vi "GeoData.vi"() -> ()   [LabVIEW 2017] (continued)
County\tH1\n51467\t19027\tWestside\tIA\tCarroll County\tH1\n51462\t19027\tScranton\tIA\tCarroll County\tH1\n50025\t19027\tAudubon\tIA\tCarroll County\tH1\n51444\t19027\tHalbur\tIA\tCarroll County\tH1\n51451\t19027\tLanesboro\tIA\tCarroll County\tH1\n51436\t19027\tBreda\tIA\tCarroll County\tH1\n51449\t19027\tLake city\tIA\tCarroll County\tH1\n51463\t19027\tTempleton\tIA\tCarroll County\tH1\n50058\t19027\tCoon rapids\tIA\tCarroll County\tH1\n51532\t19029\tElliott\tIA\tCass County\tH1\n50853\t19029\tMassena\tIA\tCass County\tH1\n50843\t19029\tCumberland\tIA\tCass County\tH1\n51552\t19029\tMarne\tIA\tCass County\tH1\n50020\t19029\tAnita\tIA\tCass County\tH1\n50042\t19029\tBrayton\tIA\tCass County\tH1\n50864\t19029\tVillisca\tIA\tCass County\tH1\n51544\t19029\tLewis\tIA\tCass County\tH1\n50022\t19029\tAtlantic\tIA\tCass County\tH1\n51577\t19029\tWalnut\tIA\tCass County\tH1\n51535\t19029\tGriswold\tIA\tCass County\tH1\n50837\t19029\tBridgewater\tIA\tCass County\tH1\n50274\t19029\tWiota\tIA\tCass County\tH1\n52253\t19031\tLisbon\tIA\tCedar County\tH1\n52720\t19031\tAtalissa\tIA\tCedar County\tH1\n52721\t19031\tBennett\tIA\tCedar County\tH1\n52776\t19031\tWest liberty\tIA\tCedar County\tH1\n52323\t19031\tOxford junction\tIA\tCedar County\tH1\n52747\t19031\tDurant\tIA\tCedar County\tH1\n52765\t19031\tNew liberty\tIA\tCedar County\tH1\n52216\t19031\tClarence\tIA\tCedar County\tH1\n52337\t19031\tStanwood\tIA\tCedar County\tH1\n52358\t19031\tWest branch\tIA\tCedar County\tH1\n52255\t19031\tLowden\tIA\tCedar County\tH1\n52333\t19031\tSolon\tIA\tCedar County\tH1\n52772\t19031\tTipton\tIA\tCedar County\tH1\n52778\t19031\tWilton\tIA\tCedar County\tH1\n52320\t19031\tOlin\tIA\tCedar County\tH1\n52760\t19031\tMoscow\tIA\tCedar County\tH1\n52306\t19031\tMechanicsville\tIA\tCedar County\tH1\n52777\t19031\tWheatland\tIA\tCedar County\tH1\n50458\t19033\tNora springs\tIA\tCerro Gordo County\tH1\n50464\t19033\tPlymouth\tIA\tCerro Gordo County\tH1\n50433\t19033\tDougherty\tIA\tCerro Gordo County\tH1\n50467\t19033\tRock falls\tIA\tCerro Gordo County\tH1\n50456\t19033\tManly\tIA\tCerro Gordo County\tH1\n50401\t19033\tMason city\tIA\tCerro Gordo County\tH1\n50469\t19033\tRockwell\tIA\tCerro Gordo County\tH1\n50428\t19033\tClear lake\tIA\tCerro Gordo County\tH1\n50477\t19033\tSwaledale\tIA\tCerro Gordo County\tH1\n50479\t19033\tThornton\tIA\tCerro Gordo County\tH1\n50475\t19033\tSheffield\tIA\tCerro Gordo County\tH1\n50438\t19033\tGarner\tIA\tCerro Gordo County\tH1\n50444\t19033\tHanlontown\tIA\tCerro Gordo County\tH1\n50468\t19033\tRockford\tIA\tCerro Gordo County\tH1\n50482\t19033\tVentura\tIA\tCerro Gordo County\tH1\n50434\t19033\tFertile\tIA\tCerro Gordo County\tH1\n50449\t19033\tKlemme\tIA\tCerro Gordo County\tH1\n50457\t19033\tMeservey\tIA\tCerro Gordo County\tH1\n50402\t19033\tMason city\tIA\tCerro Gordo County\tH1\n51047\t19035\tPeterson\tIA\tCherokee County\tH1\n51046\t19035\tPaullina\tIA\tCherokee County\tH1\n51020\t19035\tGalva\tIA\tCherokee County\tH1\n51048\t19035\tPierson\tIA\tCherokee County\tH1\n51005\t19035\tAurelia\tIA\tCherokee County\tH1\n51002\t19035\tAlta\tIA\tCherokee County\tH1\n51049\t19035\tQuimby\tIA\tCherokee County\tH1\n51037\t19035\tMeriden\tIA\tCherokee County\tH1\n51035\t19035\tMarcus\tIA\tCherokee County\tH1\n51061\t19035\tWashta\tIA\tCherokee County\tH1\n51012\t19035\tCherokee\tIA\tCherokee County\tH1\n51014\t19035\tCleghorn\tIA\tCherokee County\tH1\n51050\t19035\tRemsen\tIA\tCherokee County\tH1\n51025\t19035\tHolstein\tIA\tCherokee County\tH1\n51029\t19035\tLarrabee\tIA\tCherokee County\tH1\n51016\t19035\tCorrectionville\tIA\tCherokee County\tH1\n51022\t19035\tGranville\tIA\tCherokee County\tH1\n51058\t19035\tSutherland\tIA\tCherokee County\tH1\n52132\t19037\tCalmar\tIA\tChickasaw County\tH1\n50645\t19037\tIonia\tIA\tChickasaw County\tH1\n50603\t19037\tAlta vista\tIA\tChickasaw County\tH1\n50659\t19037\tNew hampton\tIA\tChickasaw County\tH1\n50674\t19037\tSumner\tIA\tChickasaw County\tH1\n50630\t19037\tFredericksburg\tIA\tChickasaw County\tH1\n50661\t19037\tNorth washington\tIA\tChickasaw County\tH1\n52144\t19037\tFort atkinson\tIA\tChickasaw County\tH1\n50616\t19037\tCharles city\tIA\tChickasaw County\tH1\n50658\t19037\tNashua\tIA\tChickasaw County\tH1\n52154\t19037\tLawler\tIA\tChickasaw County\tH1\n52171\t19037\tWaucoma\tIA\tChickasaw County\tH1\n50222\t19039\tPeru\tIA\tClarke County\tH1\n50108\t19039\tGrand river\tIA\tClarke County\tH1\n50257\t19039\tTruro\tIA\tClarke County\tH1\n50254\t19039\tThayer\tIA\tClarke County\tH1\n50275\t19039\tWoodburn\tIA\tClarke County\tH1\n50123\t19039\tHumeston\tIA\tClarke County\tH1\n50213\t19039\tOsceola\tIA\tClarke County\tH1\n50264\t19039\tWeldon\tIA\tClarke County\tH1\n50151\t19039\tLucas\tIA\tClarke County\tH1\n50149\t19039\tLorimor\tIA\tClarke County\tH1\n50210\t19039\tNew virginia\tIA\tClarke County\tH1\n50174\t19039\tMurray\tIA\tClarke County\tH1\n51047\t19041\tPeterson\tIA\tClay County\tH1\n51343\t19041\tGreenville\tIA\tClay County\tH1\n50554\t19041\tLaurens\tIA\tClay County\tH1\n51357\t19041\tRoyal\tIA\tClay County\tH1\n51338\t19041\tEverly\tIA\tClay County\tH1\n50565\t19041\tMarathon\tIA\tClay County\tH1\n51346\t19041\tHartley\tIA\tClay County\tH1\n51351\t19041\tMilford\tIA\tClay County\tH1\n51358\t19041\tRuthven\tIA\tClay County\tH1\n51366\t19041\tWebb\tIA\tClay County\tH1\n50515\t19041\tAyrshire\tIA\tClay County\tH1\n51333\t19041\tDickens\tIA\tClay County\tH1\n51341\t19041\tGillett grove\tIA\tClay County\tH1\n51301\t19041\tSpencer\tIA\tClay County\tH1\n51364\t19041\tTerril\tIA\tClay County\tH1\n51340\t19041\tFostoria\tIA\tClay County\tH1\n50585\t19041\tSioux rapids\tIA\tClay County\tH1\n51033\t19041\tLinn grove\tIA\tClay County\tH1\n51058\t19041\tSutherland\tIA\tClay County\tH1\n52035\t19043\tColesburg\tIA\tClayton County\tH1\n52047\t19043\tFarmersburg\tIA\tClayton County\tH1\n52169\t19043\tWadena\tIA\tClayton County\tH1\n52158\t19043\tMarquette\tIA\tClayton County\tH1\n52043\t19043\tElkader\tIA\tClayton County\tH1\n52141\t19043\tElgin\tIA\tClayton County\tH1\n52052\t19043\tGuttenberg\tIA\tClayton County\tH1\n52162\t19043\tPostville\tIA\tClayton County\tH1\n52066\t19043\tNorth buena vista\tIA\tClayton County\tH1\n52076\t19043\tStrawberry point\tIA\tClayton County\tH1\n52048\t19043\tGarber\tIA\tClayton County\tH1\n52053\t19043\tHoly cross\tIA\tClayton County\tH1\n52044\t19043\tElkport\tIA\tClayton County\tH1\n52159\t19043\tMonona\tIA\tClayton County\tH1\n52157\t19043\tMc gregor\tIA\tClayton County\tH1\n50606\t19043\tArlington\tIA\tClayton County\tH1\n52073\t19043\tSherrill\tIA\tClayton County\tH1\n52135\t19043\tClermont\tIA\tClayton County\tH1\n52072\t19043\tSaint olaf\tIA\tClayton County\tH1\n52156\t19043\tLuana\tIA\tClayton County\tH1\n52049\t19043\tGarnavillo\tIA\tClayton County\tH1\n52042\t19043\tEdgewood\tIA\tClayton County\tH1\n52077\t19043\tVolga\tIA\tClayton County\tH1\n52050\t19043\tGreeley\tIA\tClayton County\tH1\n52069\t19045\tPreston\tIA\tClinton County\tH1\n52207\t19045\tBaldwin\tIA\tClinton County\tH1\n52750\t19045\tGoose lake\tIA\tClinton County\tH1\n52730\t19045\tCamanche\tIA\tClinton County\tH1\n52771\t19045\tTeeds grove\tIA\tClinton County\tH1\n52323\t19045\tOxford junction\tIA\tClinton County\tH1\n52742\t19045\tDe witt\tIA\tClinton County\tH1\n52745\t19045\tDixon\tIA\tClinton County\tH1\n52060\t19045\tMaquoketa\tIA\tClinton County\tH1\n52727\t19045\tBryant\tIA\tClinton County\tH1\n52701\t19045\tAndover\tIA\tClinton County\tH1\n52757\t19045\tLow moor\tIA\tClinton County\tH1\n52070\t19045\tSabula\tIA\tClinton County\tH1\n52064\t19045\tMiles\tIA\tClinton County\tH1\n52756\t19045\tLong grove\tIA\tClinton County\tH1\n52309\t19045\tMonmouth\tIA\tClinton County\tH1\n52774\t19045\tWelton\tIA\tClinton County\tH1\n52254\t19045\tLost nation\tIA\tClinton County\tH1\n52732\t19045\tClinton\tIA\tClinton County\tH1\n52731\t19045\tCharlotte\tIA\tClinton County\tH1\n52729\t19045\tCalamus\tIA\tClinton County\tH1\n52037\t19045\tDelmar\tIA\tClinton County\tH1\n52777\t19045\tWheatland\tIA\tClinton County\tH1\n52751\t19045\tGrand mound\tIA\tClinton County\tH1\n51006\t19047\tBattle creek\tIA\tCrawford County\tH1\n51458\t19047\tOdebolt\tIA\tCrawford County\tH1\n51466\t19047\tWall lake\tIA\tCrawford County\tH1\n51465\t19047\tVail\tIA\tCrawford County\tH1\n51441\t19047\tDeloit\tIA\tCrawford County\tH1\n51527\t19047\tDefiance\tIA\tCrawford County\tH1\n51461\t19047\tSchleswig\tIA\tCrawford County\tH1\n51432\t19047\tAspinwall\tIA\tCrawford County\tH1\n51460\t19047\tRicketts\tIA\tCrawford County\tH1\n51455\t19047\tManning\tIA\tCrawford County\tH1\n51034\t19047\tMapleton\tIA\tCrawford County\tH1\n51467\t19047\tWestside\tIA\tCrawford County\tH1\n51529\t19047\tDunlap\tIA\tCrawford County\tH1\n51439\t19047\tCharter oak\tIA\tCrawford County\tH1\n51442\t19047\tDenison\tIA\tCrawford County\tH1\n51454\t19047\tManilla\tIA\tCrawford County\tH1\n51528\t19047\tDow city\tIA\tCrawford County\tH1\n51520\t19047\tArion\tIA\tCrawford County\tH1\n51448\t19047\tKiron\tIA\tCrawford County\tH1\n51444\t19047\tHalbur\tIA\tCrawford County\tH1\n51019\t19047\tDanbury\tIA\tCrawford County\tH1\n51060\t19047\tUte\tIA\tCrawford County\tH1\n51436\t19047\tBreda\tIA\tCrawford County\tH1\n50063\t19049\tDallas center\tIA\tDallas County\tH1\n50220\t19049\tPerry\tIA\tDallas County\tH1\n50109\t19049\tGranger\tIA\tDallas County\tH1\n50233\t19049\tRedfield\tIA\tDallas County\tH1\n50235\t19049\tRippey\tIA\tDallas County\tH1\n50146\t19049\tLinden\tIA\tDallas County\tH1\n50039\t19049\tBouton\tIA\tDallas County\tH1\n50167\t19049\tMinburn\tIA\tDallas County\tH1\n50261\t19049\tVan meter\tIA\tDallas County\tH1\n50263\t19049\tWaukee\tIA\tDallas County\tH1\n50061\t19049\tCumming\tIA\tDallas County\tH1\n50069\t19049\tDe soto\tIA\tDallas County\tH1\n50070\t19049\tDexter\tIA\tDallas County\tH1\n50325\t19049\tClive\tIA\tDallas County\tH1\n50128\t19049\tJamaica\tIA\tDallas County\tH1\n50003\t19049\tAdel\tIA\tDallas County\tH1\n50156\t19049\tMadrid\tIA\tDallas County\tH1\n50066\t19049\tDawson\tIA\tDallas County\tH1\n50216\t19049\tPanora\tIA\tDallas County\tH1\n50276\t19049\tWoodward\tIA\tDallas County\tH1\n50111\t19049\tGrimes\tIA\tDallas County\tH1\n50323\t19049\tUrbandale\tIA\tDallas County\tH1\n50277\t19049\tYale\tIA\tDallas County\tH1\n50072\t19049\tEarlham\tIA\tDallas County\tH1\n50038\t19049\tBooneville\tIA\tDallas County\tH1\n50266\t19049\tWest des moines\tIA\tDallas County\tH1\n52560\t19051\tFloris\tIA\tDavis County\tH1\n52570\t19051\tMilton\tIA\tDavis County\tH1\n52584\t19051\tPulaski\tIA\tDavis County\tH1\n52551\t19051\tDouds\tIA\tDavis County\tH1\n52552\t19051\tDrakesville\tIA\tDavis County\tH1\n52536\t19051\tBlakesburg\tIA\tDavis County\tH1\n52588\t19051\tSelma\tIA\tDavis County\tH1\n52554\t19051\tEldon\tIA\tDavis County\tH1\n52572\t19051\tMoulton\tIA\tDavis County\tH1\n52537\t19051\tBloomfield\tIA\tDavis County\tH1\n52594\t19051\tUnionville\tIA\tDavis County\tH1\n50108\t19053\tGrand river\tIA\tDecatur County\tH1\n50147\t19053\tLineville\tIA\tDecatur County\tH1\n50067\t19053\tDecatur\tIA\tDecatur County\tH1\n50140\t19053\tLamoni\tIA\tDecatur County\tH1\n50065\t19053\tDavis city\tIA\tDecatur County\tH1\n50123\t19053\tHumeston\tIA\tDecatur County\tH1\n50264\t19053\tWeldon\tIA\tDecatur County\tH1\n50262\t19053\tVan wert\tIA\tDecatur County\tH1\n50133\t19053\tKellerton\tIA\tDecatur County\tH1\n50103\t19053\tGarden grove\tIA\tDecatur County\tH1\n50144\t19053\tLeon\tIA\tDecatur County\tH1\n52065\t19055\tNew vienna\tIA\tDelaware County\tH1\n52035\t19055\tColesburg\tIA\tDelaware County\tH1\n52237\t19055\tHopkinton\tIA\tDelaware County\tH1\n52057\t19055\tManchester\tIA\tDelaware County\tH1\n52223\t19055\tDelhi\tIA\tDelaware County\tH1\n52330\t19055\tRyan\tIA\tDelaware County\tH1\n50650\t19055\tLamont\tIA\tDelaware County\tH1\n52036\t19055\tDelaware\tIA\tDelaware County\tH1\n52041\t19055\tEarlville\tIA\tDelaware County\tH1\n52076\t19055\tStrawberry point\tIA\tDelaware County\tH1\n52310\t19055\tMonticello\tIA\tDelaware County\tH1\n52038\t19055\tDundee\tIA\tDelaware County\tH1\n52078\t19055\tWorthington\tIA\tDelaware County\tH1\n50654\t19055\tMasonville\tIA\tDelaware County\tH1\n52040\t19055\tDyersville\tIA\tDelaware County\tH1\n52042\t19055\tEdgewood\tIA\tDelaware County\tH1\n52218\t19055\tCoggon\tIA\tDelaware County\tH1\n52050\t19055\tGreeley\tIA\tDelaware County\tH1\n52640\t19057\tMorning sun\tIA\tDes Moines County\tH1\n52646\t19057\tOakville\tIA\tDes Moines County\tH1\n52623\t19057\tDanville\tIA\tDes Moines County\tH1\n52638\t19057\tMiddletown\tIA\tDes Moines County\tH1\n52601\t19057\tBurlington\tIA\tDes Moines County\tH1\n52650\t19057\tSperry\tIA\tDes Moines County\tH1\n52655\t19057\tWest burlington\tIA\tDes Moines County\tH1\n52637\t19057\tMediapolis\tIA\tDes Moines County\tH1\n52645\t19057\tNew london\tIA\tDes Moines County\tH1\n52644\t19057\tMount union\tIA\tDes Moines County\tH1\n52658\t19057\tWever\tIA\tDes Moines County\tH1\n52660\t19057\tYarmouth\tIA\tDes Moines County\tH1\n51347\t19059\tLake park\tIA\tDickinson County\tH1\n51355\t19059\tOkoboji\tIA\tDickinson County\tH1\n51338\t19059\tEverly\tIA\tDickinson County\tH1\n51351\t19059\tMilford\tIA\tDickinson County\tH1\n51331\t19059\tArnolds park\tIA\tDickinson County\tH1\n51333\t19059\tDickens\tIA\tDickinson County\tH1\n51301\t19059\tSpencer\tIA\tDickinson County\tH1\n51345\t19059\tHarris\tIA\tDickinson County\tH1\n51364\t19059\tTerril\tIA\tDickinson County\tH1\n51360\t19059\tSpirit lake\tIA\tDickinson County\tH1\n51334\t19059\tEstherville\tIA\tDickinson County\tH1\n51363\t19059\tSuperior\tIA\tDickinson County\tH1\n52033\t19061\tCascade\tIA\tDubuque County\tH1\n52065\t19061\tNew vienna\tIA\tDubuque County\tH1\n52054\t19061\tLa motte\tIA\tDubuque County\tH1\n52002\t19061\tDubuque\tIA\tDubuque County\tH1\n52003\t19061\tDubuque\tIA\tDubuque County\tH1\n52039\t19061\tDurango\tIA\tDubuque County\tH1\n52045\t19061\tEpworth\tIA\tDubuque County\tH1\n52237\t19061\tHopkinton\tIA\tDubuque County\tH1\n52079\t19061\tZwingle\tIA\tDubuque County\tH1\n52056\t19061\tLuxemburg\tIA\tDubuque County\tH1\n52046\t19061\tFarley\tIA\tDubuque County\tH1\n52052\t19061\tGuttenberg\tIA\tDubuque County\tH1\n52066\t19061\tNorth buena vista\tIA\tDubuque County\tH1\n52053\t19061\tHoly cross\tIA\tDubuque County\tH1\n52099\t19061\tDubuque\tIA\tDubuque County\tH1\n52032\t19061\tBernard\tIA\tDubuque County\tH1\n52073\t19061\tSherrill\tIA\tDubuque County\tH1\n52078\t19061\tWorthington\tIA\tDubuque County\tH1\n52001\t19061\tDubuque\tIA\tDubuque County\tH1\n52068\t19061\tPeosta\tIA\tDubuque County\tH1\n52031\t19061\tBellevue\tIA\tDubuque County\tH1\n52040\t19061\tDyersville\tIA\tDubuque County\tH1\n52004\t19061\tDubuque\tIA\tDubuque County\tH1\n51365\t19063\tWallingford\tIA\tEmmet County\tH1\n50514\t19063\tArmstrong\tIA\tEmmet County\tH1\n50578\t19063\tRingsted\tIA\tEmmet County\tH1\n51342\t19063\tGraettinger\tIA\tEmmet County\tH1\n50539\t19063\tFenton\tIA\tEmmet County\tH1\n51364\t19063\tTerril\tIA\tEmmet County\tH1\n51334\t19063\tEstherville\tIA\tEmmet County\tH1\n50531\t19063\tDolliver\tIA\tEmmet County\tH1\n50655\t19065\tMaynard\tIA\tFayette County\tH1\n50662\t19065\tOelwein\tIA\tFayette County\tH1\n50681\t19065\tWestgate\tIA\tFayette County\tH1\n52147\t19065\tHawkeye\tIA\tFayette County\tH1\n52169\t19065\tWadena\tIA\tFayette County\tH1\n52141\t19065\tElgin\tIA\tFayette County\tH1\n52164\t19065\tRandalia\tIA\tFayette County\tH1\n50650\t19065\tLamont\tIA\tFayette County\tH1\n52161\t19065\tOssian\tIA\tFayette County\tH1\n52175\t19065\tWest union\tIA\tFayette County\tH1\n52162\t19065\tPostville\tIA\tFayette County\tH1\n50674\t19065\tSumner\tIA\tFayette County\tH1\n52076\t19065\tStrawberry point\tIA\tFayette County\tH1\n50664\t19065\tOran\tIA\tFayette County\tH1\n50629\t19065\tFairbank\tIA\tFayette County\tH1\n52142\t19065\tFayette\tIA\tFayette County\tH1\n50606\t19065\tArlington\tIA\tFayette County\tH1\n52133\t19065\tCastalia\tIA\tFayette County\tH1\n52135\t19065\tClermont\tIA\tFayette County\tH1\n52144\t19065\tFort atkinson\tIA\tFayette County\tH1\n50607\t19065\tAurora\tIA\tFayette County\tH1\n50671\t19065\tStanley\tIA\tFayette County\tH1\n52171\t19065\tWaucoma\tIA\tFayette County\tH1\n52166\t19065\tSaint lucas\tIA\tFayette County\tH1\n50458\t19067\tNora springs\tIA\tFloyd County\tH1\n50433\t19067\tDougherty\tIA\tFloyd County\tH1\n50461\t19067\tOsage\tIA\tFloyd County\tH1\n50636\t19067\tGreene\tIA\tFloyd County\tH1\n50653\t19067\tMarble rock\tIA\tFloyd County\tH1\n50620\t19067\tColwell\tIA\tFloyd County\tH1\n50645\t19067\tIonia\tIA\tFloyd County\tH1\n50471\t19067\tRudd\tIA\tFloyd County\tH1\n50619\t19067\tClarksville\tIA\tFloyd County\tH1\n50468\t19067\tRockford\tIA\tFloyd County\tH1\n50435\t19067\tFloyd\tIA\tFloyd County\tH1\n50460\t19067\tOrchard\tIA\tFloyd County\tH1\n50616\t19067\tCharles city\tIA\tFloyd County\tH1\n50658\t19067\tNashua\tIA\tFloyd County\tH1\n50071\t19069\tDows\tIA\tFranklin County\tH1\n50433\t19069\tDougherty\tIA\tFranklin County\tH1\n50625\t19069\tDumont\tIA\tFranklin County\tH1\n50633\t19069\tGeneva\tIA\tFranklin County\tH1\n50126\t19069\tIowa falls\tIA\tFranklin County\tH1\n50479\t19069\tThornton\tIA\tFranklin County\tH1\n50605\t19069\tAredale\tIA\tFranklin County\tH1\n50475\t19069\tSheffield\tIA\tFranklin County\tH1\n50470\t19069\tRowan\tIA\tFranklin County\tH1\n50452\t19069\tLatimer\tIA\tFranklin County\tH1\n50601\t19069\tAckley\tIA\tFranklin County\tH1\n50006\t19069\tAlden\tIA\tFranklin County\tH1\n50420\t19069\tAlexander\tIA\tFranklin County\tH1\n50427\t19069\tChapin\tIA\tFranklin County\tH1\n50441\t19069\tHampton\tIA\tFranklin County\tH1\n50457\t19069\tMeservey\tIA\tFranklin County\tH1\n50041\t19069\tBradford\tIA\tFranklin County\tH1\n50227\t19069\tPopejoy\tIA\tFranklin County\tH1\n50431\t19069\tCoulter\tIA\tFranklin County\tH1\n51647\t19071\tNorthboro\tIA\tFremont County\tH1\n51551\t19071\tMalvern\tIA\tFremont County\tH1\n51640\t19071\tHamburg\tIA\tFremont County\tH1\n51648\t19071\tPercival\tIA\tFremont County\tH1\n51650\t19071\tRiverton\tIA\tFremont County\tH1\n51603\t19071\tShenandoah\tIA\tFremont County\tH1\n51601\t19071\tShenandoah\tIA\tFremont County\tH1\n51654\t19071\tThurman\tIA\tFremont County\tH1\n51649\t19071\tRandolph\tIA\tFremont County\tH1\n51653\t19071\tTabor\tIA\tFremont County\tH1\n51639\t19071\tFarragut\tIA\tFremont County\tH1\n51652\t19071\tSidney\tIA\tFremont County\tH1\n51645\t19071\tImogene\tIA\tFremont County\tH1\n50220\t19073\tPerry\tIA\tGreene County\tH1\n50543\t19073\tGowrie\tIA\tGreene County\tH1\n50064\t19073\tDana\tIA\tGreene County\tH1\n50235\t19073\tRippey\tIA\tGreene County\tH1\n50026\t19073\tBagley\tIA\tGreene County\tH1\n51453\t19073\tLohrville\tIA\tGreene County\tH1\n50050\t19073\tChurdan\tIA\tGreene County\tH1\n51443\t19073\tGlidden\tIA\tGreene County\tH1\n50029\t19073\tBayard\tIA\tGreene County\tH1\n50128\t19073\tJamaica\tIA\tGreene County\tH1\n51462\t19073\tScranton\tIA\tGreene County\tH1\n50544\t19073\tHarcourt\tIA\tGreene County\tH1\n50217\t19073\tPaton\tIA\tGreene County\tH1\n50107\t19073\tGrand junction\tIA\tGreene County\tH1\n51449\t19073\tLake city\tIA\tGreene County\tH1\n50129\t19073\tJefferson\tIA\tGreene County\tH1\n50058\t19073\tCoon rapids\tIA\tGreene County\tH1\n50059\t19073\tCooper\tIA\tGreene County\tH1\n50638\t19075\tGrundy center\tIA\tGrundy County\tH1\n50148\t19075\tLiscomb\tIA\tGrundy County\tH1\n50621\t19075\tConrad\tIA\tGrundy County\tH1\n50613\t19075\tCedar falls\tIA\tGrundy County\tH1\n50657\t19075\tMorrison\tIA\tGrundy County\tH1\n50672\t19075\tSteamboat rock\tIA\tGrundy County\tH1\n50669\t19075\tReinbeck\tIA\tGrundy County\tH1\n50609\t19075\tBeaman\tIA\tGrundy County\tH1\n50269\t19075\tWhitten\tIA\tGrundy County\tH1\n50673\t19075\tStout\tIA\tGrundy County\tH1\n50601\t19075\tAckley\tIA\tGrundy County\tH1\n50680\t19075\tWellsburg\tIA\tGrundy County\tH1\n50665\t19075\tParkersburg\tIA\tGrundy County\tH1\n50624\t19075\tDike\tIA\tGrundy County\tH1\n50642\t19075\tHolland\tIA\tGrundy County\tH1\n50258\t19075\tUnion\tIA\tGrundy County\tH1\n50627\t19075\tEldora\tIA\tGrundy County\tH1\n50604\t19075\tAplington\tIA\tGrundy County\tH1\n50660\t19075\tNew hartford\tIA\tGrundy County\tH1\n50643\t19075\tHudson\tIA\tGrundy County\tH1\n50002\t19077\tAdair\tIA\tGuthrie County\tH1\n50076\t19077\tExira\tIA\tGuthrie County\tH1\n50233\t19077\tRedfield\tIA\tGuthrie County\tH1\n50115\t19077\tGuthrie center\tIA\tGuthrie County\tH1\n50146\t19077\tLinden\tIA\tGuthrie County\tH1\n50048\t19077\tCasey\tIA\tGuthrie County\tH1\n50026\t19077\tBagley\tIA\tGuthrie County\tH1\n50250\t19077\tStuart\tIA\tGuthrie County\tH1\n50070\t19077\tDexter\tIA\tGuthrie County\tH1\n50020\t19077\tAnita\tIA\tGuthrie County\tH1\n50029\t19077\tBayard\tIA\tGuthrie County\tH1\n50128\t19077\tJamaica\tIA\tGuthrie County\tH1\n50216\t19077\tPanora\tIA\tGuthrie County\tH1\n50164\t19077\tMenlo\tIA\tGuthrie County\tH1\n50277\t19077\tYale\tIA\tGuthrie County\tH1\n50129\t19077\tJefferson\tIA\tGuthrie County\tH1\n50058\t19077\tCoon rapids\tIA\tGuthrie County\tH1\n50236\t19079\tRoland\tIA\tHamilton County\tH1\n50230\t19079\tRadcliffe\tIA\tHamilton County\tH1\n50246\t19079\tStanhope\tIA\tHamilton County\tH1\n50231\t19079\tRandall\tIA\tHamilton County\tH1\n50034\t19079\tBlairsburg\tIA\tHamilton County\tH1\n50132\t19079\tKamrar\tIA\tHamilton County\tH1\n50595\t19079\tWebster city\tIA\tHamilton County\tH1\n50599\t19079\tWoolstock\tIA\tHamilton County\tH1\n50036\t19079\tBoone\tIA\tHamilton County\tH1\n50249\t19079\tStratford\tIA\tHamilton County\tH1\n50271\t19079\tWilliams\tIA\tHamilton County\tH1\n50006\t19079\tAlden\tIA\tHamilton County\tH1\n50075\t19079\tEllsworth\tIA\tHamilton County\tH1\n50248\t19079\tStory city\tIA\tHamilton County\tH1\n50532\t19079\tDuncombe\tIA\tHamilton County\tH1\n50130\t19079\tJewell\tIA\tHamilton County\tH1\n50447\t19081\tKanawha\tIA\tHancock County\tH1\n50483\t19081\tWesley\tIA\tHancock County\tH1\n50438\t19081\tGarner\tIA\tHancock County\tH1\n50423\t19081\tBritt\tIA\tHancock County\tH1\n50482\t19081\tVentura\tIA\tHancock County\tH1\n50439\t19081\tGoodell\tIA\tHancock County\tH1\n50484\t19081\tWoden\tIA\tHancock County\tH1\n50421\t19081\tBelmond\tIA\tHancock County\tH1\n50432\t19081\tCrystal lake\tIA\tHancock County\tH1\n50436\t19081\tForest city\tIA\tHancock County\tH1\n50449\t19081\tKlemme\tIA\tHancock County\tH1\n50457\t19081\tMeservey\tIA\tHancock County\tH1\n50430\t19081\tCorwith\tIA\tHancock County\tH1\n50206\t19083\tNew providence\tIA\tHardin County\tH1\n50259\t19083\tGifford\tIA\tHardin County\tH1\n50230\t19083\tRadcliffe\tIA\tHardin County\tH1\n50126\t19083\tIowa falls\tIA\tHardin County\tH1\n50122\t19083\tHubbard\tIA\tHardin County\tH1\n50672\t19083\tSteamboat rock\tIA\tHardin County\tH1\n50271\t19083\tWilliams\tIA\tHardin County\tH1\n50269\t19083\tWhitten\tIA\tHardin County\tH1\n50601\t19083\tAckley\tIA\tHardin County\tH1\n50006\t19083\tAlden\tIA\tHardin County\tH1\n50102\t19083\tGarden city\tIA\tHardin County\tH1\n50258\t19083\tUnion\tIA\tHardin County\tH1\n50154\t19083\tMc callsburg\tIA\tHardin County\tH1\n50627\t19083\tEldora\tIA\tHardin County\tH1\n50227\t19083\tPopejoy\tIA\tHardin County\tH1\n51550\t19085\tMagnolia\tIA\tHarrison County\tH1\n51557\t19085\tMondamin\tIA\tHarrison County\tH1\n51564\t19085\tPisgah\tIA\tHarrison County\tH1\n51563\t19085\tPersia\tIA\tHarrison County\tH1\n51579\t19085\tWoodbine\tIA\tHarrison County\tH1\n51545\t19085\tLittle sioux\tIA\tHarrison County\tH1\n51555\t19085\tMissouri valley\tIA\tHarrison County\tH1\n51562\t19085\tPanama\tIA\tHarrison County\tH1\n51523\t19085\tBlencoe\tIA\tHarrison County\tH1\n51529\t19085\tDunlap\tIA\tHarrison County\tH1\n51565\t19085\tPortsmouth\tIA\tHarrison County\tH1\n51530\t19085\tEarling\tIA\tHarrison County\tH1\n51559\t19085\tNeola\tIA\tHarrison County\tH1\n51556\t19085\tModale\tIA\tHarrison County\tH1\n51546\t19085\tLogan\tIA\tHarrison County\tH1\n51570\t19085\tShelby\tIA\tHarrison County\tH1\n51558\t19085\tMoorhead\tIA\tHarrison County\tH1\n52656\t19087\tWest point\tIA\tHenry County\tH1\n52641\t19087\tMount pleasant\tIA\tHenry County\tH1\n52659\t19087\tWinfield\tIA\tHenry County\tH1\n52621\t19087\tCrawfordsville\tIA\tHenry County\tH1\n52647\t19087\tOlds\tIA\tHenry County\tH1\n52620\t19087\tBonaparte\tIA\tHenry County\tH1\n52652\t19087\tSwedesburg\tIA\tHenry County\tH1\n52630\t19087\tHillsboro\tIA\tHenry County\tH1\n52623\t19087\tDanville\tIA\tHenry County\tH1\n52635\t19087\tLockridge\tIA\tHenry County\tH1\n52637\t19087\tMediapolis\tIA\tHenry County\tH1\n52645\t19087\tNew london\tIA\tHenry County\tH1\n52644\t19087\tMount union\tIA\tHenry County\tH1\n52649\t19087\tSalem\tIA\tHenry County\tH1\n52654\t19087\tWayland\tIA\tHenry County\tH1\n50628\t19089\tElma\tIA\tHoward County\tH1\n52132\t19089\tCalmar\tIA\tHoward County\tH1\n52163\t19089\tProtivin\tIA\tHoward County\tH1\n50603\t19089\tAlta vista\tIA\tHoward County\tH1\n50466\t19089\tRiceville\tIA\tHoward County\tH1\n50659\t19089\tNew hampton\tIA\tHoward County\tH1\n52136\t19089\tCresco\tIA\tHoward County\tH1\n52134\t19089\tChester\tIA\tHoward County\tH1\n52155\t19089\tLime springs\tIA\tHoward County\tH1\n52154\t19089\tLawler\tIA\tHoward County\tH1\n52171\t19089\tWaucoma\tIA\tHoward County\tH1\n50519\t19091\tBode\tIA\tHumboldt County\tH1\n50548\t19091\tHumboldt\tIA\tHumboldt County\tH1\n50570\t19091\tOttosen\tIA\tHumboldt County\tH1\n50516\t19091\tBadger\tIA\tHumboldt County\tH1\n50558\t19091\tLivermore\tIA\tHumboldt County\tH1\n50560\t19091\tLu verne\tIA\tHumboldt County\tH1\n50520\t19091\tBradgate\tIA\tHumboldt County\tH1\n50541\t19091\tGilmore city\tIA\tHumboldt County\tH1\n50542\t19091\tGoldfield\tIA\tHumboldt County\tH1\n50577\t19091\tRenwick\tIA\tHumboldt County\tH1\n50524\t19091\tClare\tIA\tHumboldt County\tH1\n50529\t19091\tDakota city\tIA\tHumboldt County\tH1\n50591\t19091\tThor\tIA\tHumboldt County\tH1\n50582\t19091\tRutland\tIA\tHumboldt County\tH1\n50533\t19091\tEagle grove\tIA\tHumboldt County\tH1\n50545\t19091\tHardy\tIA\tHumboldt County\tH1\n50597\t19091\tWest bend\tIA\tHumboldt County\tH1\n50430\t19091\tCorwith\tIA\tHumboldt County\tH1\n51006\t19093\tBattle creek\tIA\tIda County\tH1\n51020\t19093\tGalva\tIA\tIda County\tH1\n51445\t19093\tIda grove\tIA\tIda County\tH1\n51461\t19093\tSchleswig\tIA\tIda County\tH1\n51431\t19093\tArthur\tIA\tIda County\tH1\n51053\t19093\tSchaller\tIA\tIda County\tH1\n51061\t19093\tWashta\tIA\tIda County\tH1\n51448\t19093\tKiron\tIA\tIda County\tH1\n51019\t19093\tDanbury\tIA\tIda County\tH1\n51025\t19093\tHolstein\tIA\tIda County\tH1\n51016\t19093\tCorrectionville\tIA\tIda County\tH1\n51018\t19093\tCushing\tIA\tIda County\tH1\n52361\t19095\tWilliamsburg\tIA\tIowa County\tH1\n50136\t19095\tKeswick\tIA\tIowa County\tH1\n52232\t19095\tHartwick\tIA\tIowa County\tH1\n52236\t19095\tHomestead\tIA\tIowa County\tH1\n52204\t19095\tAmana\tIA\tIowa County\tH1\n52222\t19095\tDeep river\tIA\tIowa County\tH1\n52355\t19095\tWebster\tIA\tIowa County\tH1\n52301\t19095\tMarengo\tIA\tIowa County\tH1\n52347\t19095\tVictor\tIA\tIowa County\tH1\n52322\t19095\tOxford\tIA\tIowa County\tH1\n52209\t19095\tBlairstown\tIA\tIowa County\tH1\n52203\t19095\tAmana\tIA\tIowa County\tH1\n52318\t19095\tNorway\tIA\tIowa County\tH1\n52221\t19095\tGuernsey\tIA\tIowa County\tH1\n52316\t19095\tNorth english\tIA\tIowa County\tH1\n52307\t19095\tMiddle amana\tIA\tIowa County\tH1\n52208\t19095\tBelle plaine\tIA\tIowa County\tH1\n52356\t19095\tWellman\tIA\tIowa County\tH1\n52334\t19095\tSouth amana\tIA\tIowa County\tH1\n52308\t19095\tMillersburg\tIA\tIowa County\tH1\n52220\t19095\tConroy\tIA\tIowa County\tH1\n52325\t19095\tParnell\tIA\tIowa County\tH1\n52251\t19095\tLadora\tIA\tIowa County\tH1\n52069\t19097\tPreston\tIA\tJackson County\tH1\n52207\t19097\tBaldwin\tIA\tJackson County\tH1\n52054\t19097\tLa motte\tIA\tJackson County\tH1\n52030\t19097\tAndrew\tIA\tJackson County\tH1\n52079\t19097\tZwingle\tIA\tJackson County\tH1\n52060\t19097\tMaquoketa\tIA\tJackson County\tH1\n52071\t19097\tSaint donatus\tIA\tJackson County\tH1\n52070\t19097\tSabula\tIA\tJackson County\tH1\n52064\t19097\tMiles\tIA\tJackson County\tH1\n52074\t19097\tSpragueville\tIA\tJackson County\tH1\n52309\t19097\tMonmouth\tIA\tJackson County\tH1\n52032\t19097\tBernard\tIA\tJackson County\tH1\n52731\t19097\tCharlotte\tIA\tJackson County\tH1\n52031\t19097\tBellevue\tIA\tJackson County\tH1\n52037\t19097\tDelmar\tIA\tJackson County\tH1\n52075\t19097\tSpringbrook\tIA\tJackson County\tH1\n50170\t19099\tMonroe\tIA\tJasper County\tH1\n50153\t19099\tLynnville\tIA\tJasper County\tH1\n50169\t19099\tMitchellville\tIA\tJasper County\tH1\n50214\t19099\tOtley\tIA\tJasper County\tH1\n50137\t19099\tKillduff\tIA\tJasper County\tH1\n50161\t19099\tMaxwell\tIA\tJasper County\tH1\n50054\t19099\tColfax\tIA\tJasper County\tH1\n50237\t19099\tRunnells\tIA\tJasper County\tH1\n50251\t19099\tSully\tIA\tJasper County\tH1\n50168\t19099\tMingo\tIA\tJasper County\tH1\n50112\t19099\tGrinnell\tIA\tJasper County\tH1\n50141\t19099\tLaurel\tIA\tJasper County\tH1\n50228\t19099\tPrairie city\tIA\tJasper County\tH1\n50234\t19099\tRhodes\tIA\tJasper County\tH1\n50127\t19099\tIra\tIA\tJasper County\tH1\n50208\t19099\tNewton\tIA\tJasper County\tH1\n50162\t19099\tMelbourne\tIA\tJasper County\tH1\n50232\t19099\tReasnor\tIA\tJasper County\tH1\n50135\t19099\tKellogg\tIA\tJasper County\tH1\n50055\t19099\tCollins\tIA\tJasper County\tH1\n50028\t19099\tBaxter\tIA\tJasper County\tH1\n50106\t19099\tGilman\tIA\tJasper County\tH1\n50242\t19099\tSearsboro\tIA\tJasper County\tH1\n52641\t19101\tMount pleasant\tIA\tJefferson County\tH1\n52585\t19101\tRichland\tIA\tJefferson County\tH1\n52533\t19101\tBatavia\tIA\tJefferson County\tH1\n52563\t19101\tHedrick\tIA\tJefferson County\tH1\n52540\t19101\tBrighton\tIA\tJefferson County\tH1\n52576\t19101\tOllie\tIA\tJefferson County\tH1\n52556\t19101\tFairfield\tIA\tJefferson County\tH1\n52580\t19101\tPackwood\tIA\tJefferson County\tH1\n52567\t19101\tLibertyville\tIA\tJefferson County\tH1\n52588\t19101\tSelma\tIA\tJefferson County\tH1\n52635\t19101\tLockridge\tIA\tJefferson County\tH1\n52554\t19101\tEldon\tIA\tJefferson County\tH1\n52535\t19101\tBirmingham\tIA\tJefferson County\tH1\n52651\t19101\tStockport\tIA\tJefferson County\tH1\n52654\t19101\tWayland\tIA\tJefferson County\tH1\n52557\t19101\tFairfield\tIA\tJefferson County\tH1\n52240\t19103\tIowa city\tIA\tJohnson County\tH1\n52247\t19103\tKalona\tIA\tJohnson County\tH1\n52253\t19103\tLisbon\tIA\tJohnson County\tH1\n52338\t19103\tSwisher\tIA\tJohnson County\tH1\n52776\t19103\tWest liberty\tIA\tJohnson County\tH1\n52322\t19103\tOxford\tIA\tJohnson County\tH1\n52242\t19103\tIowa city\tIA\tJohnson County\tH1\n52235\t19103\tHills\tIA\tJohnson County\tH1\n52244\t19103\tIowa city\tIA\tJohnson County\tH1\n52203\t19103\tAmana\tIA\tJohnson County\tH1\n52404\t19103\tCedar rapids\tIA\tJohnson County\tH1\n52766\t19103\tNichols\tIA\tJohnson County\tH1\n52241\t19103\tCoralville\tIA\tJohnson County\tH1\n52340\t19103\tTiffin\tIA\tJohnson County\tH1\n52358\t19103\tWest branch\tIA\tJohnson County\tH1\n52227\t19103\tEly\tIA\tJohnson County\tH1\n52755\t19103\tLone tree\tIA\tJohnson County\tH1\n52245\t19103\tIowa city\tIA\tJohnson County\tH1\n52228\t19103\tFairfax\tIA\tJohnson County\tH1\n52333\t19103\tSolon\tIA\tJohnson County\tH1\n52317\t19103\tNorth liberty\tIA\tJohnson County\tH1\n52356\t19103\tWellman\tIA\tJohnson County\tH1\n52246\t19103\tIowa city\tIA\tJohnson County\tH1\n52314\t19103\tMount vernon\tIA\tJohnson County\tH1\n52327\t19103\tRiverside\tIA\tJohnson County\tH1\n52325\t19103\tParnell\tIA\tJohnson County\tH1\n52243\t19103\tIowa city\tIA\tJohnson County\tH1\n52033\t19105\tCascade\tIA\tJones County\tH1\n52253\t19105\tLisbon\tIA\tJones County\tH1\n52212\t19105\tCenter junction\tIA\tJones County\tH1\n52205\t19105\tAnamosa\tIA\tJones County\tH1\n52237\t19105\tHopkinton\tIA\tJones County\tH1\n52321\t19105\tOnslow\tIA\tJones County\tH1\n52323\t19105\tOxford junction\tIA\tJones County\tH1\n52252\t19105\tLangworthy\tIA\tJones County\tH1\n52216\t19105\tClarence\tIA\tJones County\tH1\n52336\t19105\tSpringville\tIA\tJones County\tH1\n52309\t19105\tMonmouth\tIA\tJones County\tH1\n52032\t19105\tBernard\tIA\tJones County\tH1\n52362\t19105\tWyoming\tIA\tJones County\tH1\n52310\t19105\tMonticello\tIA\tJones County\tH1\n52320\t19105\tOlin\tIA\tJones County\tH1\n52306\t19105\tMechanicsville\tIA\tJones County\tH1\n52305\t19105\tMartelle\tIA\tJones County\tH1\n52218\t19105\tCoggon\tIA\tJones County\tH1\n52312\t19105\tMorley\tIA\tJones County\tH1\n50268\t19107\tWhat cheer\tIA\tKeokuk County\tH1\n52585\t19107\tRichland\tIA\tKeokuk County\tH1\n50104\t19107\tGibson\tIA\tKeokuk County\tH1\n50136\t19107\tKeswick\tIA\tKeokuk County\tH1\n52563\t19107\tHedrick\tIA\tKeokuk County\tH1\n52550\t19107\tDelta\tIA\tKeokuk County\tH1\n52335\t19107\tSouth english\tIA\tKeokuk County\tH1\n52562\t19107\tHayesville\tIA\tKeokuk County\tH1\n52586\t19107\tRose hill\tIA\tKeokuk County\tH1\n52561\t19107\tFremont\tIA\tKeokuk County\tH1\n52355\t19107\tWebster\tIA\tKeokuk County\tH1\n52568\t19107\tMartinsburg\tIA\tKeokuk County\tH1\n52501\t19107\tOttumwa\tIA\tKeokuk County\tH1\n52576\t19107\tOllie\tIA\tKeokuk County\tH1\n52580\t19107\tPackwood\tIA\tKeokuk County\tH1\n52316\t19107\tNorth english\tIA\tKeokuk County\tH1\n52356\t19107\tWellman\tIA\tKeokuk County\tH1\n52248\t19107\tKeota\tIA\tKeokuk County\tH1\n52591\t19107\tSigourney\tIA\tKeokuk County\tH1\n52231\t19107\tHarper\tIA\tKeokuk County\tH1\n50255\t19107\tThornburg\tIA\tKeokuk County\tH1\n50480\t19109\tTitonka\tIA\tKossuth County\tH1\n50517\t19109\tBancroft\tIA\tKossuth County\tH1\n50519\t19109\tBode\tIA\tKossuth County\tH1\n50570\t19109\tOttosen\tIA\tKossuth County\tH1\n50424\t19109\tBuffalo center\tIA\tKossuth County\tH1\n50514\t19109\tArmstrong\tIA\tKossuth County\tH1\n50483\t19109\tWesley\tIA\tKossuth County\tH1\n50558\t19109\tLivermore\tIA\tKossuth County\tH1\n50560\t19109\tLu verne\tIA\tKossuth County\tH1\n50539\t19109\tFenton\tIA\tKossuth County\tH1\n50511\t19109\tAlgona\tIA\tKossuth County\tH1\n50522\t19109\tBurt\tIA\tKossuth County\tH1\n50559\t19109\tLone rock\tIA\tKossuth County\tH1\n50484\t19109\tWoden\tIA\tKossuth County\tH1\n50598\t19109\tWhittemore\tIA\tKossuth County\tH1\n50451\t19109\tLakota\tIA\tKossuth County\tH1\n50556\t19109\tLedyard\tIA\tKossuth County\tH1\n50590\t19109\tSwea city\tIA\tKossuth County\tH1\n50597\t19109\tWest bend\tIA\tKossuth County\tH1\n50430\t19109\tCorwith\tIA\tKossuth County\tH1\n52656\t19111\tWest point\tIA\tLee County\tH1\n52632\t19111\tKeokuk\tIA\tLee County\tH1\n52648\t19111\tPilot grove\tIA\tLee County\tH1\n52627\t19111\tFort madison\tIA\tLee County\tH1\n52630\t19111\tHillsboro\tIA\tLee County\tH1\n52625\t19111\tDonnellson\tIA\tLee County\tH1\n52619\t19111\tArgyle\tIA\tLee County\tH1\n52626\t19111\tFarmington\tIA\tLee County\tH1\n52639\t19111\tMontrose\tIA\tLee County\tH1\n52658\t19111\tWever\tIA\tLee County\tH1\n52657\t19111\tSaint paul\tIA\tLee County\tH1\n52624\t19111\tDenmark\tIA\tLee County\tH1\n52631\t19111\tHoughton\tIA\tLee County\tH1\n52649\t19111\tSalem\tIA\tLee County\tH1\n52213\t19113\tCenter point\tIA\tLinn County\tH1\n52302\t19113\tMarion\tIA\tLinn County\tH1\n52253\t19113\tLisbon\tIA\tLinn County\tH1\n52205\t19113\tAnamosa\tIA\tLinn County\tH1\n52405\t19113\tCedar rapids\tIA\tLinn County\tH1\n52332\t19113\tShellsburg\tIA\tLinn County\tH1\n52338\t19113\tSwisher\tIA\tLinn County\tH1\n52352\t19113\tWalker\tIA\tLinn County\tH1\n52406\t19113\tCedar rapids\tIA\tLinn County\tH1\n52409\t19113\tCedar rapids\tIA\tLinn County\tH1\n52498\t19113\tCedar rapids\tIA\tLinn County\tH1\n52233\t19113\tHiawatha\tIA\tLinn County\tH1\n52404\t19113\tCedar rapids\tIA\tLinn County\tH1\n52351\t19113\tWalford\tIA\tLinn County\tH1\n52410\t19113\tCedar rapids\tIA\tLinn County\tH1\n52202\t19113\tAlburnett\tIA\tLinn County\tH1\n52214\t19113\tCentral city\tIA\tLinn County\tH1\n52336\t19113\tSpringville\tIA\tLinn County\tH1\n52324\t19113\tPalo\tIA\tLinn County\tH1\n52227\t19113\tEly\tIA\tLinn County\tH1\n52408\t19113\tCedar rapids\tIA\tLinn County\tH1\n52499\t19113\tCedar rapids\tIA\tLinn County\tH1\n52228\t19113\tFairfax\tIA\tLinn County\tH1\n52333\t19113\tSolon\tIA\tLinn County\tH1\n52402\t19113\tCedar rapids\tIA\tLinn County\tH1\n52310\t19113\tMonticello\tIA\tLinn County\tH1\n52401\t19113\tCedar rapids\tIA\tLinn County\tH1\n52344\t19113\tTroy mills\tIA\tLinn County\tH1\n52403\t19113\tCedar rapids\tIA\tLinn County\tH1\n52314\t19113\tMount vernon\tIA\tLinn County\tH1\n52411\t19113\tCedar rapids\tIA\tLinn County\tH1\n52305\t19113\tMartelle\tIA\tLinn County\tH1\n52218\t19113\tCoggon\tIA\tLinn County\tH1\n52341\t19113\tToddville\tIA\tLinn County\tH1\n52328\t19113\tRobins\tIA\tLinn County\tH1\n52219\t19113\tPrairieburg\tIA\tLinn County\tH1\n52659\t19115\tWinfield\tIA\tLouisa County\tH1\n52621\t19115\tCrawfordsville\tIA\tLouisa County\tH1\n52737\t19115\tColumbus city\tIA\tLouisa County\tH1\n52752\t19115\tGrandview\tIA\tLouisa County\tH1\n52640\t19115\tMorning sun\tIA\tLouisa County\tH1\n52646\t19115\tOakville\tIA\tLouisa County\tH1\n52761\t19115\tMuscatine\tIA\tLouisa County\tH1\n52739\t19115\tConesville\tIA\tLouisa County\tH1\n52738\t19115\tColumbus junction\tIA\tLouisa County\tH1\n52201\t19115\tAinsworth\tIA\tLouisa County\tH1\n52754\t19115\tLetts\tIA\tLouisa County\tH1\n52755\t19115\tLone tree\tIA\tLouisa County\tH1\n52637\t19115\tMediapolis\tIA\tLouisa County\tH1\n52653\t19115\tWapello\tIA\tLouisa County\tH1\n52644\t19115\tMount union\tIA\tLouisa County\tH1\n52327\t19115\tRiverside\tIA\tLouisa County\tH1\n50060\t19117\tCorydon\tIA\tLucas County\tH1\n50049\t19117\tChariton\tIA\tLucas County\tH1\n50238\t19117\tRussell\tIA\tLucas County\tH1\n50275\t19117\tWoodburn\tIA\tLucas County\tH1\n50123\t19117\tHumeston\tIA\tLucas County\tH1\n50139\t19117\tLacona\tIA\tLucas County\tH1\n50272\t19117\tWilliamson\tIA\tLucas County\tH1\n50151\t19117\tLucas\tIA\tLucas County\tH1\n50068\t19117\tDerby\tIA\tLucas County\tH1\n52569\t19117\tMelrose\tIA\tLucas County\tH1\n51201\t19119\tSheldon\tIA\tLyon County\tH1\n51242\t19119\tLester\tIA\tLyon County\tH1\n51243\t19119\tLittle rock\tIA\tLyon County\tH1\n51234\t19119\tBoyden\tIA\tLyon County\tH1\n51235\t19119\tDoon\tIA\tLyon County\tH1\n51237\t19119\tGeorge\tIA\tLyon County\tH1\n51246\t19119\tRock rapids\tIA\tLyon County\tH1\n51239\t19119\tHull\tIA\tLyon County\tH1\n51247\t19119\tRock valley\tIA\tLyon County\tH1\n51240\t19119\tInwood\tIA\tLyon County\tH1\n51230\t19119\tAlvord\tIA\tLyon County\tH1\n51249\t19119\tSibley\tIA\tLyon County\tH1\n51232\t19119\tAshton\tIA\tLyon County\tH1\n51241\t19119\tLarchwood\tIA\tLyon County\tH1\n50222\t19121\tPeru\tIA\tMadison County\tH1\n50218\t19121\tPatterson\tIA\tMadison County\tH1\n50155\t19121\tMacksburg\tIA\tMadison County\tH1\n50273\t19121\tWinterset\tIA\tMadison County\tH1\n50257\t19121\tTruro\tIA\tMadison County\tH1\n50858\t19121\tOrient\tIA\tMadison County\tH1\n50229\t19121\tProle\tIA\tMadison County\tH1\n50240\t19121\tSaint charles\tIA\tMadison County\tH1\n50261\t19121\tVan meter\tIA\tMadison County\tH1\n50061\t19121\tCumming\tIA\tMadison County\tH1\n50069\t19121\tDe soto\tIA\tMadison County\tH1\n50070\t19121\tDexter\tIA\tMadison County\tH1\n50801\t19121\tCreston\tIA\tMadison County\tH1\n50211\t19121\tNorwalk\tIA\tMadison County\tH1\n50149\t19121\tLorimor\tIA\tMadison County\tH1\n50072\t19121\tEarlham\tIA\tMadison County\tH1\n50033\t19121\tBevington\tIA\tMadison County\tH1\n50038\t19121\tBooneville\tIA\tMadison County\tH1\n50210\t19121\tNew virginia\tIA\tMadison County\tH1\n50174\t19121\tMurray\tIA\tMadison County\tH1\n50268\t19123\tWhat cheer\tIA\tMahaska County\tH1\n52553\t19123\tEddyville\tIA\tMahaska County\tH1\n50153\t19123\tLynnville\tIA\tMahaska County\tH1\n50104\t19123\tGibson\tIA\tMahaska County\tH1\n52543\t19123\tCedar\tIA\tMahaska County\tH1\n50219\t19123\tPella\tIA\tMahaska County\tH1\n52550\t19123\tDelta\tIA\tMahaska County\tH1\n50143\t19123\tLeighton\tIA\tMahaska County\tH1\n52586\t19123\tRose hill\tIA\tMahaska County\tH1\n52561\t19123\tFremont\tIA\tMahaska County\tH1\n50251\t19123\tSully\tIA\tMahaska County\tH1\n52501\t19123\tOttumwa\tIA\tMahaska County\tH1\n50044\t19123\tBussey\tIA\tMahaska County\tH1\n52534\t19123\tBeacon\tIA\tMahaska 
